vi "SP Check Calibration From INI File.vi"(7 "Paramters to Measure":T4[](array[typedef]) {"Channel" min=1 max=99 step=1; "Parameter"."Stimulus Port" min=1 step=1; "Parameter"."Response Port" min=1 step=1}, 8 "error in (no error)":errorcluster, 11 "Requested Stimulus":T1={"Use Instrument Settings"=FALSE, "Blank Frequencies"=FALSE, "Sweep Type"=enum."Linear", "Sweep"={"Fstart"=500.0, "Fstop"=1500.0, "Units"=enum."MHz", "Points"=201}, "Power (dBm)"=999.0, "IFBW (Hz)"=-1.0, "Sweep Time (s)"=-1.0, "Calibration"={"State"=FALSE, "String"=""}} {"Sweep Time (s)" format="%.3g"}) -> (0 "error out":errorcluster, 1 "Check Instrument":bool, 3 "Stimulus Out":T1={"Use Instrument Settings"=FALSE, "Blank Frequencies"=FALSE, "Sweep Type"=enum."Linear", "Sweep"={"Fstart"=500.0, "Fstop"=1500.0, "Units"=enum."MHz", "Points"=201}, "Power (dBm)"=999.0, "IFBW (Hz)"=-1.0, "Sweep Time (s)"=-1.0, "Calibration"={"State"=FALSE, "String"=""}} {"Sweep Time (s)" format="%.3g"}, 5 "Paramters to Measure Out":T4[](array[typedef]) {"Channel" min=1 max=99 step=1; "Parameter"."Stimulus Port" min=1 step=1; "Parameter"."Response Port" min=1 step=1})   [LabVIEW 2011]
uses:
  TypeDefs/SP Parameter to Measure.ctl
  TypeDefs/SP Parameter.ctl
  TypeDefs/SP Calibration State.ctl
  TypeDefs/SP Measurement Format.ctl
  TypeDefs/SP Stimulus Parameters.ctl
  TypeDefs/SP Frequency Units.ctl
  <vilib>/Utility/config.llb/Read Key (String).vi
  <vilib>/Utility/config.llb/NI_LVConfig.lvlib
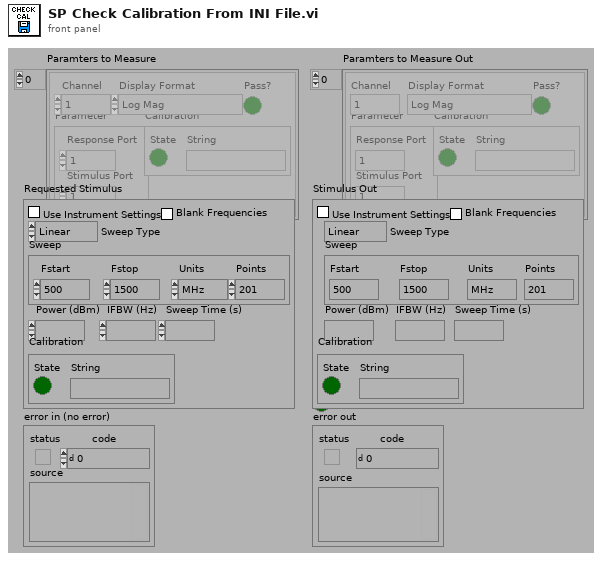
[diagram p1: front panel]
types:
  T1 = typedef "SP Stimulus Parameters.ctl" = cluster{"Use Instrument Settings":bool, "Blank Frequencies":bool, "Sweep Type":enum32{"Linear", "Logarithmic", "List", "Power", "CW"}, "Sweep":cluster{"Fstart":dbl, "Fstop":dbl, "Units":T2, "Points":i32}, "Power (dBm)":dbl, "IFBW (Hz)":dbl, "Sweep Time (s)":dbl, "Calibration":T3}
  T2 = typedef "SP Frequency Units.ctl" = enum16{"Hz", "kHz", "MHz", "GHz", "Points"}
  T3 = typedef "SP Calibration State.ctl" = cluster{"State":bool, "String":string}
  T4 = typedef "SP Parameter to Measure.ctl" = cluster{"Channel":i8, "Parameter":T5, "Calibration":T3, "Display Format":T6, "Pass?":bool}
  T5 = typedef "SP Parameter.ctl" = cluster{"Stimulus Port":i8, "Response Port":i8}
  T6 = typedef "SP Measurement Format.ctl" = enum32{"Log Mag", "Phase", "Delay", "Smith (R+jX)", "Polar (Re/Im)", "Linear Mag", "SWR", "Real", "Imaginary", "Smith (Lin/Phase)", "Smith (Log/Phase)", "Smith (Real/Imag)", "Smith (G+jB)", "Polar (Lin/Phase)", "Polar (Log/Phase)", "Expanded Phase", "Positive Phase", "Inverted Smith", "Unwrapped Phase", "Power Out", "Power In", "Linear Mag/Phase", "Log Mag/Phase", "Real/Imaginary"}
  T7 = typedef "NI_LVConfig.lvlib/Config Data RefNum.ctl" = refnum<k1>
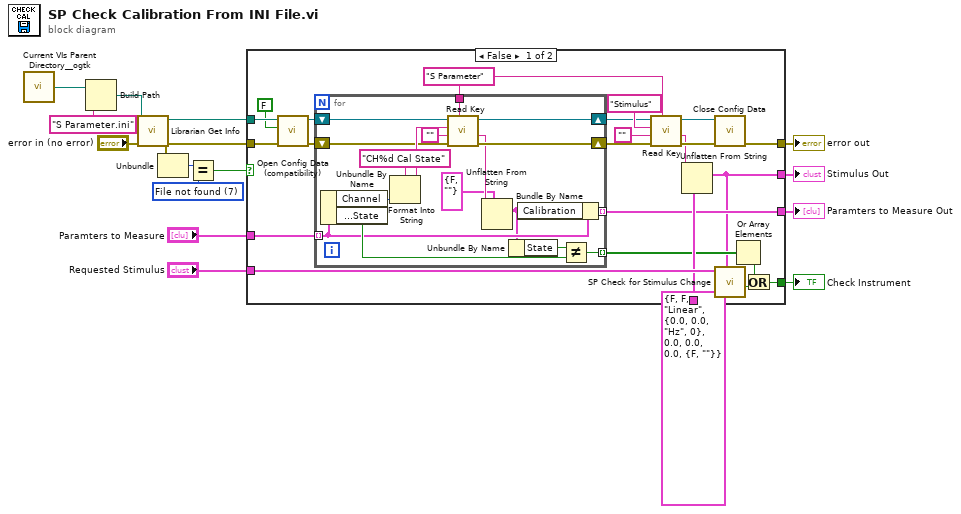
[diagram p0: block diagram]
diagram:
  w12 = 7 items=["No error", "Argument error", "Memory is full", "Out of zone", "End of file", "File already open", "Generic file I/O error", "File not found", "File permission error", "Disk is full", "Duplicate path", "Too many files open", "System feature not enabled", "Resource file not found", "Cannot add resource", "Resource not found", "Image not found", "Image memory error", "Pen does not exist", "Config type invalid", "Config token not found", "Config parse error", "Config memory error", "Bad external code format", "Bad external code offset", "External code not present", "Null window", "Destroy window error", "Null menu", "Print aborted", "Bad print record", "Print driver error", "Windows error during printing", "Memory error during printing", "Print dialog error", "Generic print error", "Invalid device refnum", "Device not found", "Device parameter error", "Device unit error", "Cannot open device", "Device call aborted", "Generic error", "Cancelled by user", "Object ID too low", "Object ID too high", "Object not in heap", "Unknown heap", "Unknown object (invalid DefProc)", "Unknown object (DefProc not in table)", "Message out of range", "Invalid (null) method", "Unknown message", "Manager call not supported", "Bad address", "Network operation in progress", "Network operation timed out", "Connection is busy", "Network attribute not supported", "Network error", "Address in use", "System out of memory", "Connection aborted", "Connection refused", "Not connected", "Already connected", "Connection closed", "Initialization error (interapplication manager)", "Bad occurrence", "Wait on unbound occurrence handler", "Occurrence queue overflow", "Datalog type conflict", "Unused", "Unrecognized type (interapplication manager)", "Memory corrupt", "Failed to make temporary DLL", "Old CIN version", "Drag socket not found", "Failed to load drop-object", "Failed to register OLE object", "Failed to release OLE object", "Format specifier type mismatch", "Unknown format specifier", "Too few format specifiers", "Too many format specifiers", "Scan failed", "Newer CIN version", "Error converting to variant", "Runtime menu error", "Password tampered", "Variant attribute not found", "Incompatible variant data type", "Event data is not available", "Event Store is not present", "Occurrence is not found", "Event Queue is not created", "Event info is not available in the type library", "Refnum passed is NULL", "Error retrieving Class GUID", "Error retrieving CoClass GUID", "Error retrieving TypeLib GUID.", "Bad built application magic bytes.", "Specific driver is different from the specific driver associated with the Logical Name.", "There is no session opened to the class driver.", "Max Error", "MAX - Error with config objects", "MAX - Error loading configuration", "MAX - Group not supported", "Singlecast connections can not send to multicast addresses.", "Multicast connections can not send to singlecast addresses.", "Specified IP address not in multicast address range.", "Attempt to write to read-only multicast connection.", "Attempt to read from write-only multicast connection.", "The buffer used to receive a datagram was smaller than the datagram itself"]
  n1 = call "Current VIs Parent Directory__ogtk.vi"() -> ("Parent Directory (+ Relative)"=w1:path)  [unwired: 5 in]
  n2 = Build Path(base path=w1, name or relative path="S Parameter.ini") -> (appended path=w15:path)
  n3 = call <vilib>:"Librarian Get Info.vi"("error in (no error)"="error in (no error)", "path"=w15) -> ("error out"=w10:errorcluster, "dup path"=w9:path)  [unwired: 8 out]
  n4 = Unbundle(w10) -> ("code"=w13:i32)  [unwired: 2 out]
  n5 = Equal?(x=w13, y=w12) -> (x = y?=w11:bool)
  n6 = case shown="False" w11 {
    selector: w11 -> [_ w57]
    tunnel: w10 -> [w39 _]
    tunnel: [w33 _] -> w7
    tunnel: w9 -> [w38 _]
    tunnel: [w37 w57] -> w8
    tunnel: "Requested Stimulus" -> [w36 _]
    tunnel: "Paramters to Measure" -> [w27 _]
    tunnel: T1 {"Use Instrument Settings"=FALSE, "Blank Frequencies"=FALSE, "Sweep Type"=enum."Linear", "Sweep"={"Fstart"=0.0, "Fstop"=0.0, "Units"=enum."Hz", "Points"=0}, "Power (dBm)"=0.0, "IFBW (Hz)"=0.0, "Sweep Time (s)"=0.0, "Calibration"={"State"=FALSE, "String"=""}} ("Stimulus") -> [w28 _]
    tunnel: [w18 _] -> w3
    tunnel: [w17 _] -> w2
    frame False {
      w20 = "S Parameter" ("name or relative path")
      n7 = call <vilib>:"Open Config Data (compatibility).vi"("error in (no error)"=w39, "create file if necessary (T)"=FALSE ("create file if necessary? (T)"), "configuration file path"=w38) -> ("error out"=w26:errorcluster, "refnum"=w25:T7)  [unwired: 6 in, 1 out]
      n8 = for {
        tunnel: w27 -> [w42] mode=indexing
        shift-right: [w52] -> w24
        shift-left: w26 -> [w53]
        shift-right: [w51] -> w23
        shift-left: w25 -> [w48]
        tunnel: [w49] -> w22 mode=indexing
        tunnel: w20 -> [w47]
        tunnel: [w41] -> w18 mode=indexing
        n9 = Unbundle By Name(w42) -> ("Channel"=w46:i8, "Calibration.State"=w44:bool)
        n10 = Format Into String(format string="CH%d Cal State", w46) -> (resulting string=w54:string)  [unwired: 2 in, 1 out]
        n11 = call-poly <vilib>:"Read Key.vi"("section"=w47, "error in (no error)"=w53, "default value"="", "key"=w54, "refnum"=w48) -> ("error out"=w52:errorcluster, "value"=w50:string, "refnum out"=w51:T7)  [unwired: 1 in, 3 out]
        n12 = Unflatten From String(type=T3 {"State"=FALSE, "String"=""} ("Calibration State"), binary string=w50) -> (value=w40:T3)  [unwired: 1 in, 4 out]
        n13 = Unbundle By Name(w40) -> ("State"=w43:bool)
        n14 = Bundle By Name(cluster=w42, "Calibration"=w40) -> (w41:T4)
        n15 = Not Equal?(x=w43, y=w44) -> (x != y?=w49:bool)
      }
      n16 = call-poly <vilib>:"Read Key.vi"("section"=w20, "error in (no error)"=w24, "default value"="", "key"="Stimulus", "refnum"=w23) -> ("error out"=w34:errorcluster, "value"=w29:string, "refnum out"=w32:T7)  [unwired: 1 in, 3 out]
      n17 = Unflatten From String(type=w28, binary string=w29) -> (value=w17:T1)  [unwired: 1 in, 4 out]
      n18 = call <vilib>:"Close Config Data.vi"("error in (no error)"=w34, "refnum"=w32) -> ("error out"=w33:errorcluster)  [unwired: 1 in, 8 out]
      n19 = call "SP Check for Stimulus Change.vi"("Current Stimulus Channel"=w17, "New Stimulus"=w36) -> ("Stimulus Changed?"=w35:bool)  [unwired: 1 in, 8 out]
      n20 = Or Array Elements(Boolean array=w22) -> (logical OR=w21:bool)
      n21 = Or(x=w21, y=w35) -> (x .or. y?=w37:bool)
    }
    frame True {
    }
  }
  "error out" <- w7
  "Check Instrument" <- w8
  "Paramters to Measure Out" <- w3
  "Stimulus Out" <- w2
